vi "controlActorSelection.vi"(8 "error in":errorcluster, 9 "Positioner in":string, 10 "axis in":u8, 11 "connection ID":refnum<k5>) -> (0 "error out":errorcluster, 2 "axis out":u8, 3 "connection ID":refnum<k5>)   [LabVIEW 2016]
panel:
  in  "Set Command":string="com.attocube.amc.control.setActorParametersByName"
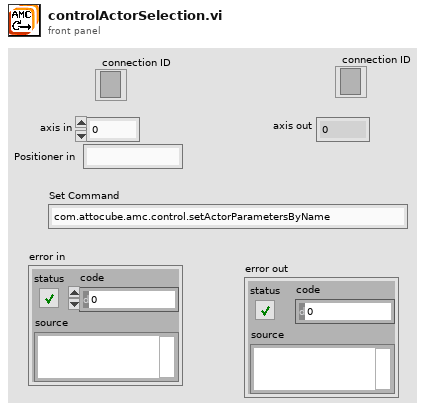
[diagram p1: front panel]
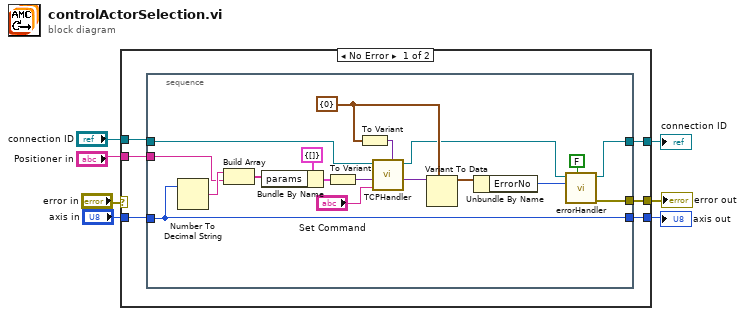
[diagram p0: block diagram]
diagram:
  n1 = case shown="No Error" "error in" {
    selector: "error in" -> [_ w32]
    tunnel: "axis in" -> [w13 w33]
    tunnel: [w8 w32] -> w6
    tunnel: [w9 w33] -> w5
    tunnel: "Positioner in" -> [w12 _]
    tunnel: [w10 w34] -> w3
    tunnel: "connection ID" -> [w11 w34]
    frame No Error {
      n2 = stacked-sequence {
        tunnel: [w14] -> w10
        tunnel: w11 -> [w22]
        tunnel: w13 -> [w18]
        tunnel: [w18] -> w9
        tunnel: [w23] -> w8
        tunnel: w12 -> [w16]
        frame #0 {
          w20 = cluster{"ErrorNo":i16} {"ErrorNo"=0} ("input cluster")
          n3 = Number To Decimal String(number=w18) -> (decimal integer string=w17:string)  [unwired: 1 in]
          n4 = Build Array(w17, w16) -> (w27:string[])
          n5 = Bundle By Name(cluster=cluster{"params":string[]} {"params"=[]} ("input cluster"), "params"=w27) -> (w28:cluster{"params":string[]})
          n6 = To Variant(anything=w28) -> (Variant=w29:variant)
          n7 = To Variant(anything=w20) -> (Variant=w21:variant)
          n8 = call "TCPHandler.vi"("result Types"=w21, "method"="Set Command", "params"=w29, "connection ID"=w22) -> ("result"=w25:variant, "connection ID"=w15:refnum<k5>)  [unwired: 5 in, 1 out]
          n9 = Variant To Data(type=w20, Variant=w25) -> (data=w30:cluster{"ErrorNo":i16})  [unwired: 1 in, 1 out]
          n10 = Unbundle By Name(w30) -> ("ErrorNo"=w31:i16)
          n11 = call "errorHandler.vi"("show popup"=FALSE, "error number"=w31, "connection ID"=w15) -> ("error out"=w23:errorcluster, "connection ID"=w14:refnum<k5>)  [unwired: 7 in]
        }
      }
    }
    frame Error {
    }
  }
  "error out" <- w6
  "axis out" <- w5
  "connection ID" <- w3
